vi "Parsing_Activation.vi"(11 "ActivationCode":string) -> (1 "使用期限":i32, 3 "MAC":string)   [LabVIEW 2018]
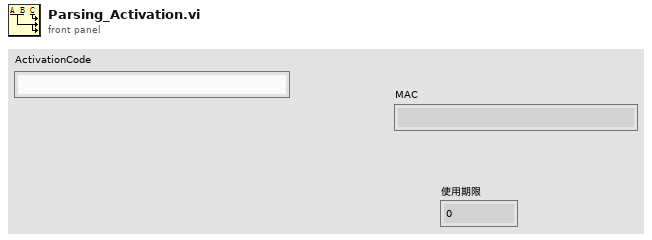
[diagram p1: front panel]
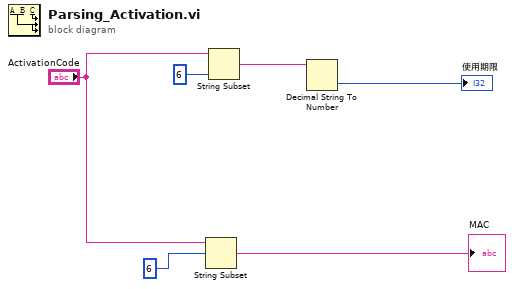
[diagram p0: block diagram]
diagram:
  n1 = String Subset(string="ActivationCode", offset (0)=6 ("偏移量(0)")) -> (substring=→"MAC":string)  [unwired: 1 in]
  n2 = String Subset(string="ActivationCode", length (rest)=6 ("长度（剩余）")) -> (substring=w4:string)  [unwired: 1 in]
  n3 = Decimal String To Number(string=w4) -> (number=→"使用期限":i32)  [unwired: 2 in, 1 out]
